vi "Index Array.vi"(3 "error in (no error)":errorcluster, 4 "index":i32, 5 "Controller Array in":refnum<class "Controller Array.lvclass">) -> (0 "error out":errorcluster, 1 "element":refnum<class "Generic Plugin.lvclass">, 2 "Controller Array out":refnum<class "Controller Array.lvclass">)   [LabVIEW 2020, in "RxnRover.lvlib" / "Controller Array.lvclass"]
uses:
  Controller Array.lvclass
  Controller/Generic Plugin.lvclass
  Controller Array.lvclass/Controller Array.ctl
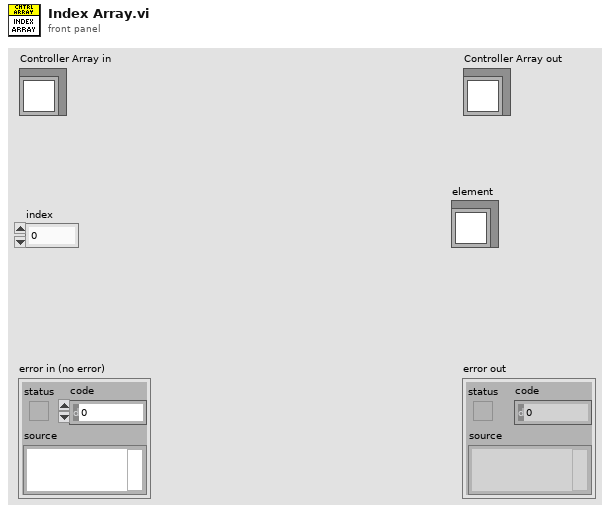
[diagram p1: front panel]
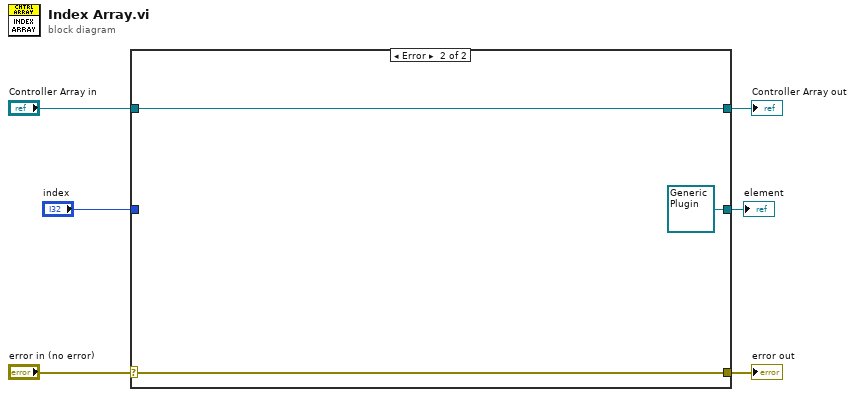
[diagram p0: block diagram]
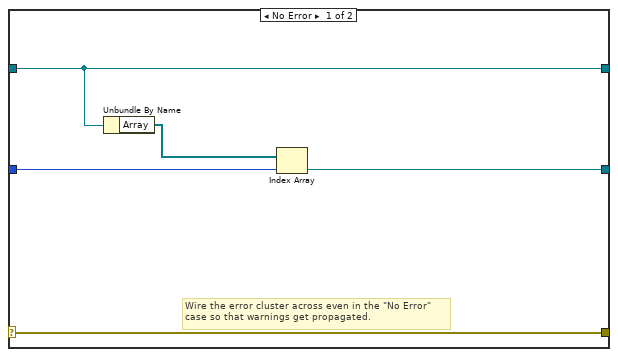
[diagram p2: hidden frame]
diagram:
  n1 = case shown="Error" "error in (no error)" {
    selector: "error in (no error)" -> [w11 w14]
    tunnel: [w11 w14] -> w5
    tunnel: [w10 w13] -> w3
    tunnel: "Controller Array in" -> [w10 w13]
    tunnel: "index" -> [w8 _]
    tunnel: [w7 refnum<class "Generic Plugin.lvclass"> refnum ("Controller.lvclass")] -> w1
    frame No Error {
      # "Wire the error cluster across even in the \"No Error\"\ncase so that warnings get propagated."
      n2 = Unbundle By Name(w10) -> ("Array"=w9:refnum<class "Generic Plugin.lvclass">[])
      n3 = Index Array(array=w9, index=w8) -> (element=w7:refnum<class "Generic Plugin.lvclass">)
    }
    frame Error {
    }
  }
  "error out" <- w5
  "Controller Array out" <- w3
  "element" <- w1
